vi "NR_ReSourceData.vi"(7 "imagrxpath":path, 8 "error in (no error)":errorcluster caption="错误输入（无错误）", 9 "tbdata":dbl[](array[numeric]), 11 "appended path":path) -> (0 "error IO":errorcluster, 3 "imagrxpathout":path)   [LabVIEW 2015]
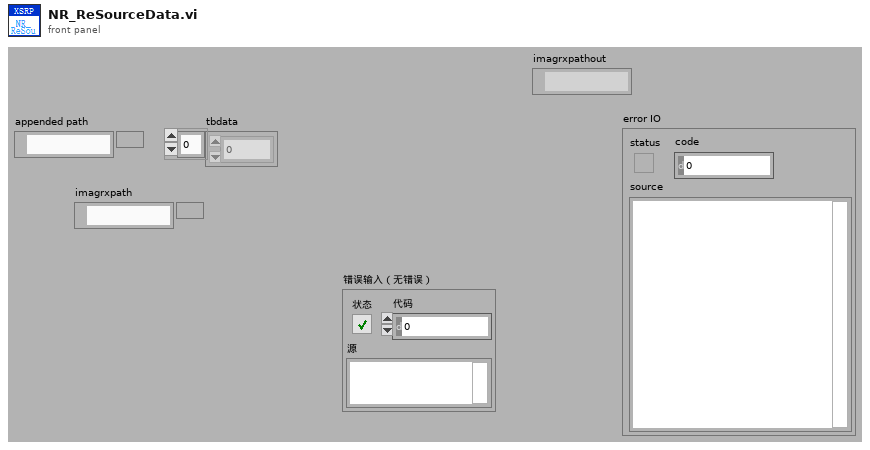
[diagram p1: front panel]
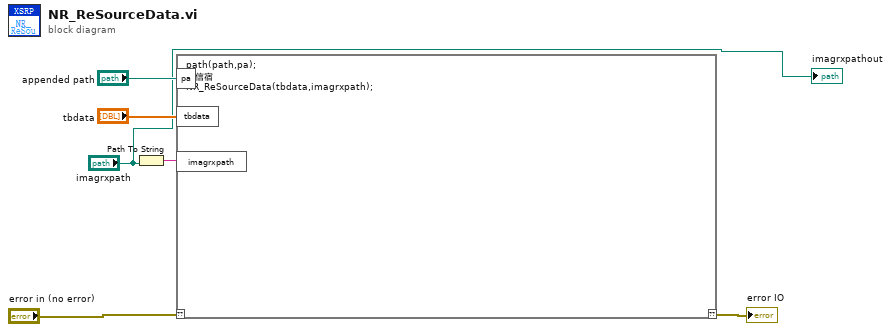
[diagram p0: block diagram]
diagram:
  n1 = Path To String(path="imagrxpath") -> (string=w2:string)
  n2 = script code="path(path,pa);\n%信宿\nNR_ReSourceData(tbdata,imagrxpath);"("??"="error in (no error)", "pa"="appended path", "tbdata"="tbdata", "imagrxpath"=w2) -> ("??"=→"error IO":errorcluster)
  "imagrxpathout" <- "imagrxpath"
